vi "AlternatingLEDs.vi"() -> ()   [LabVIEW 2014]
panel:
  in  "stop":bool
  in  "Boolean":bool
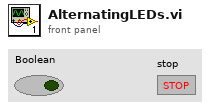
[diagram p1: front panel]
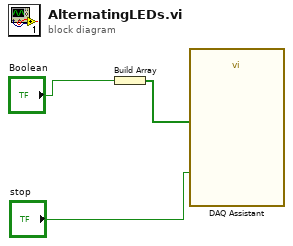
[diagram p0: block diagram]
diagram:
  n1 = Build Array("Boolean") -> (w2:bool[])
  n2 = call "DAQ Assistant"("data"=w2, "stop (T)"="stop") -> ()  [unwired: 16 in, 2 out]
